vi "Return Project Memory.vi"(11 "Full Documentation":T2) -> (3 "Memory":T1)   [LabVIEW 2023, in "VIDoc Printer.lvlib" / "VIDoc Printer.lvclass"]
doc: "Returns the full project memory give the Full Documentation."
uses:
  VIDoc Printer.lvclass
  VIDoc Printer.lvclass/VIDoc Printer.ctl
  Parsing/TypeDefs/Memory Size Cluster.ctl
  Parsing/VIDoc Parsing.lvlib
  Parsing/GUI Documentation/GUI Documentation.lvclass
  Parsing/Library Documentation/Library Documentation.lvclass
  Parsing/Class Documentation/Class Documentation.lvclass
  Parsing/Project Documentation/Project Documentation.lvclass
  Parsing/Interface Documenation/Interface Documenation.lvclass
  Parsing/TypeDefs/Full Documentation Info.ctl
  Parsing/LLB Documentation/LLB Documentation.lvclass
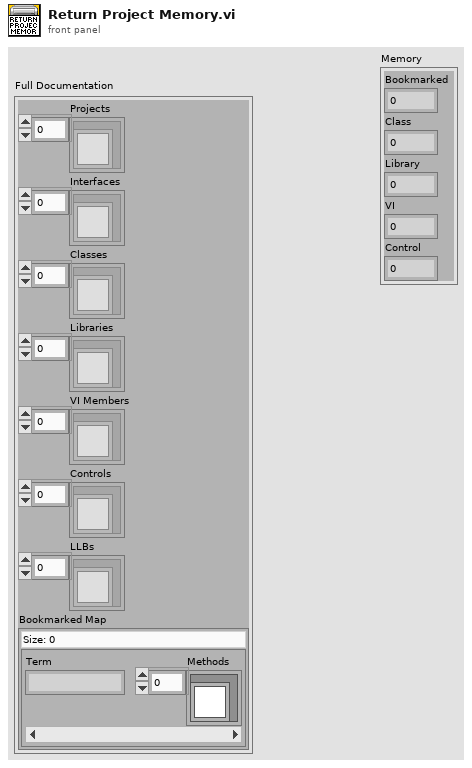
[diagram p1: front panel]
types:
  T1 = typedef "VIDoc Parsing.lvlib/Memory Size Cluster.ctl" = cluster{"Bookmarked":dbl, "Class":dbl, "Library":dbl, "VI":dbl, "Control":dbl}
  T2 = typedef "VIDoc Parsing.lvlib/Full Documentation Info.ctl" = cluster{"Projects":refnum<class "Project Documentation.lvclass">[], "Interfaces":refnum<class "Interface Documenation.lvclass">[], "Classes":refnum<class "Class Documentation.lvclass">[], "Libraries":refnum<class "Library Documentation.lvclass">[], "VI Members":refnum<class "GUI Documentation.lvclass">[], "Controls":refnum<class "GUI Documentation.lvclass">[], "LLBs":refnum<class "LLB Documentation.lvclass">[], "Bookmarked Map":map{string, refnum<class "GUI Documentation.lvclass">[]}}
  T3 = map{string, refnum<class "GUI Documentation.lvclass">[]}
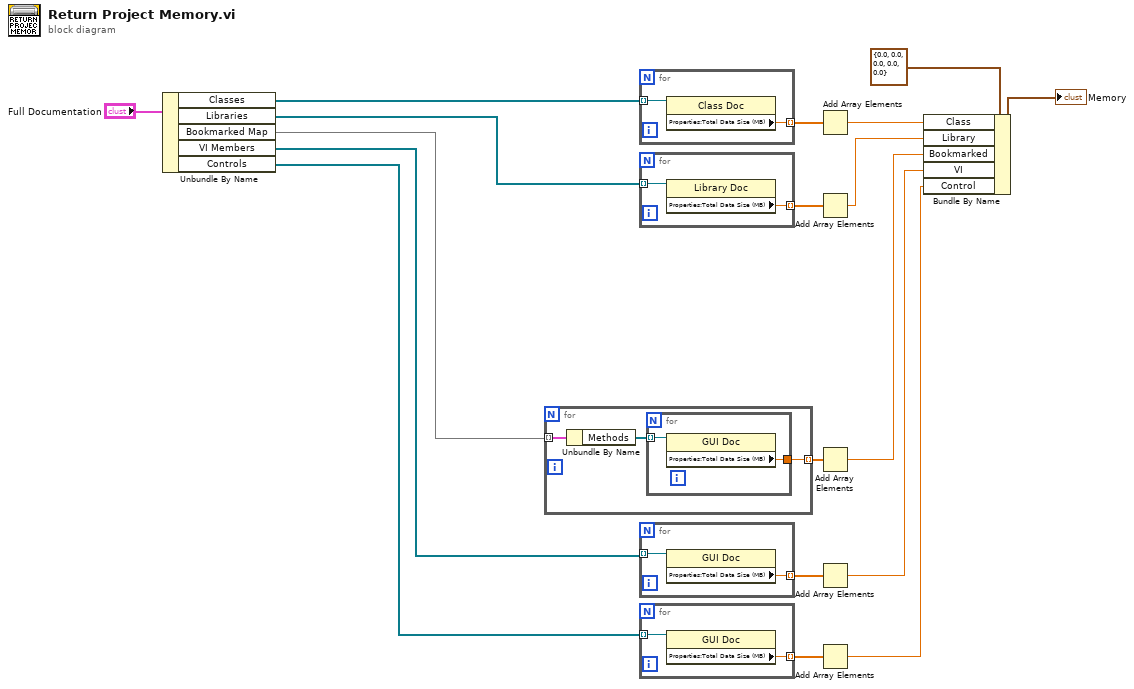
[diagram p0: block diagram]
diagram:
  n1 = Unbundle By Name("Full Documentation") -> ("Classes"=w17:refnum<class "Class Documentation.lvclass">[], "Libraries"=w8:refnum<class "Library Documentation.lvclass">[], "Bookmarked Map"=w7:T3, "VI Members"=w6:refnum<class "GUI Documentation.lvclass">[], "Controls"=w5:refnum<class "GUI Documentation.lvclass">[])
  n2 = for {
    tunnel: w7 -> [w21] mode=indexing
    tunnel: [w20] -> w11 mode=indexing
    n3 = Unbundle By Name(w21) -> ("Methods"=w19:refnum<class "GUI Documentation.lvclass">[])
    n4 = for {
      tunnel: w19 -> [w23] mode=indexing
      tunnel: [w22] -> w20
      n5 = property class="GUI Doc"(reference=w23) -> ("Properties:Total Data Size (MB)"=w22:dbl)  [unwired: 1 in, 2 out]
    }
  }
  n6 = for {
    tunnel: w17 -> [w25] mode=indexing
    tunnel: [w24] -> w16 mode=indexing
    n7 = property class="Class Doc"(reference=w25) -> ("Properties:Total Data Size (MB)"=w24:dbl)  [unwired: 1 in, 2 out]
  }
  n8 = for {
    tunnel: w8 -> [w27] mode=indexing
    tunnel: [w26] -> w12 mode=indexing
    n9 = property class="Library Doc"(reference=w27) -> ("Properties:Total Data Size (MB)"=w26:dbl)  [unwired: 1 in, 2 out]
  }
  n10 = for {
    tunnel: w6 -> [w29] mode=indexing
    tunnel: [w28] -> w10 mode=indexing
    n11 = property class="GUI Doc"(reference=w29) -> ("Properties:Total Data Size (MB)"=w28:dbl)  [unwired: 1 in, 2 out]
  }
  n12 = for {
    tunnel: w5 -> [w31] mode=indexing
    tunnel: [w30] -> w9 mode=indexing
    n13 = property class="GUI Doc"(reference=w31) -> ("Properties:Total Data Size (MB)"=w30:dbl)  [unwired: 1 in, 2 out]
  }
  n14 = Add Array Elements(numeric array=w16) -> (sum=w13:dbl)
  n15 = Add Array Elements(numeric array=w12) -> (sum=w4:dbl)
  n16 = Add Array Elements(numeric array=w11) -> (sum=w3:dbl)
  n17 = Add Array Elements(numeric array=w10) -> (sum=w2:dbl)
  n18 = Add Array Elements(numeric array=w9) -> (sum=w1:dbl)
  n19 = Bundle By Name(cluster=T1 {"Bookmarked"=0.0, "Class"=0.0, "Library"=0.0, "VI"=0.0, "Control"=0.0} ("Memory"), "Class"=w13, "Library"=w4, "Bookmarked"=w3, "VI"=w2, "Control"=w1) -> (→"Memory":T1)
